vi "Get_MultiVar_Values.vi"(8 "error in (no error)":errorcluster, 10 "varNames":string[](array[string]), 11 "mupExpr in":refnum<data-value>) -> (0 "error out":errorcluster, 2 "Values":dbl[](array[numeric]), 3 "mupExpr out":refnum<data-value>)   [LabVIEW 2015, in "mupExpr.lvclass"]
doc: "Lookup multiple variable values by name."
uses:
  mupExpr.lvclass
  mupExpr.lvclass/mupExpr.ctl
  <vilib>/Utility/error.llb/Error Cluster From Error Code.vi
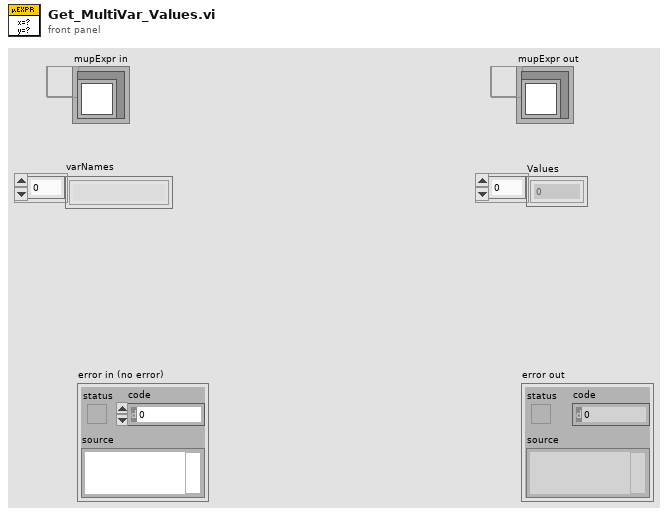
[diagram p1: front panel]
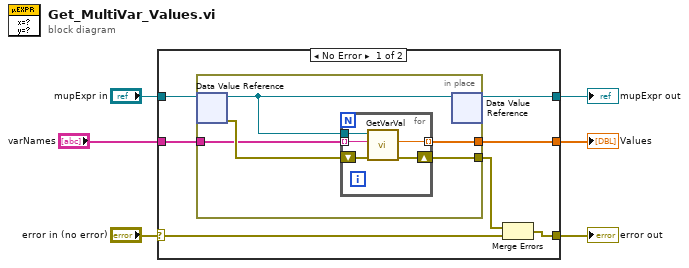
[diagram p0: block diagram]
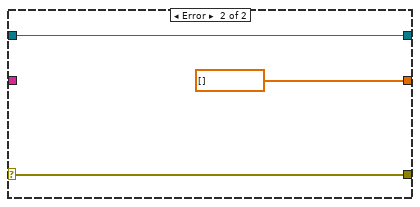
[diagram p2: hidden frame]
diagram:
  n1 = case shown="No Error" "error in (no error)" {
    selector: "error in (no error)" -> [w10 w26]
    tunnel: [w8 w26] -> w5
    tunnel: [w11 w25] -> w3
    tunnel: "mupExpr in" -> [w12 w25]
    tunnel: [w13 dbl[] [] ("pd")] -> w2
    tunnel: "varNames" -> [w7 _]
    frame No Error {
      n2 = in-place {
        in-place-border: [w18] -> w9
        in-place-border: [w17] -> w13
        in-place-border: w7 -> [w15]
        n3 = in-place-dvr #1(w12) -> (w14:refnum<class "mupExpr.lvclass">, w16:errorcluster)
        n4 = for {
          tunnel: [w19] -> w17 mode=indexing
          shift-right: [w20] -> w18
          shift-left: w16 -> [w21]
          tunnel: w15 -> [w22] mode=indexing
          tunnel: w14 -> [w23]
          n5 = call "GetVarVal.vi"("error in (no error)"=w21, "varName"=w22, "muExpr in"=w23) -> ("error out"=w20:errorcluster, "varValue"=w19:dbl)  [unwired: 6 in, 1 out]
        }
        n6 = in-place-dvr #1(w14) -> (w11:refnum<data-value>)  [unwired: 1 out]
      }
      n7 = Merge Errors(w9, w10) -> (w8:errorcluster)
    }
    frame Error {
    }
  }
  "error out" <- w5
  "mupExpr out" <- w3
  "Values" <- w2
